vi "HPCNC CONTROL.vi"() -> ()   [LabVIEW 2014]
uses:
  SubVIs/HPCNC.lvlib
  <vilib>/Native 3D Graph/xcontrol/3DPC_SurfacePlot.xctl
  <vilib>/Instr/_visa.llb/VISA Configure Serial Port (Instr).vi
panel:
  out "New package":string
  in  "Enable":bool=TRUE
  in  "Stop":bool
  in  "Auto/Manual":bool=TRUE
  in  "Serial COM port":refnum<visa-resource-name>="COM4"
  in  "Pause":bool caption="Blank Button"
  in  "Start":bool caption="Blank Button"
  in  "RESET":bool caption="Blank Button"
  in  "HOME":bool caption="Blank Button"
  out "Check sum":bool=TRUE
  out "STATUS":string="Idle"
  out "Zm":string="0.000"
  out "Ym":string="-21.164"
  out "Xm":string="148.408"
  in  "Ys0":bool
  in  "Zs0":bool
  in  "Xs0":bool
  out "Za":string="0.000"
  out "Ya":string="0.000"
  out "Xa":string="0.000"
  in  "Enable Graph":bool
  in  "Clear Button":bool
  out "3D Graph":refnum<class "Base Datatype.lvclass">[](xcontrol)
  in  "JOG FR":i8(slide)=50 scale=0.0..100.0
  in  "Z-":bool caption="Blank Button"
  in  "Z+":bool caption="Blank Button"
  in  "Y-":bool caption="Blank Button"
  in  "Y+":bool caption="Blank Button"
  in  "X-":bool caption="Blank Button"
  in  "X+":bool caption="Blank Button"
  out "MANUAL":bool
  out "Current feed rate":string="0"
  in  "AUTO FR":i8(slide)=50 scale=0.0..100.0
  in  "G Code":string="G01X0Y0Z0F1000"
  in  "Send G code":bool caption="Blank Button"
  out "AUTOMATIC":bool=TRUE
  out "Receive data":string="\u001a0164<Id,MPos:148.408,-21.164,0.000,0.000,WPos:0.000,0.000,0.000,-3.500,Ln:0,F:0.,Fp:100,S:0.,Sp:100,SP:0,CL:0,MI:0,AS:1,JT:0,JM:0,Hi:0,AL:0,BC:458,CS:07\r\n"
  # "STATUS"
  # "MACHINE POSITION"
  # "X:"
  # "Y:"
  # "Z:"
  # "ABSOLUTE POSITION"
  # "X:"
  # "Y:"
  # "Z:"
  # "SIMULATION 3D"
  # "JOG"
  # "JOG FEED(%)"
  # "CMD:"
  # "CURRENT FEED RATE:"
  # "FEED RATE(%)"
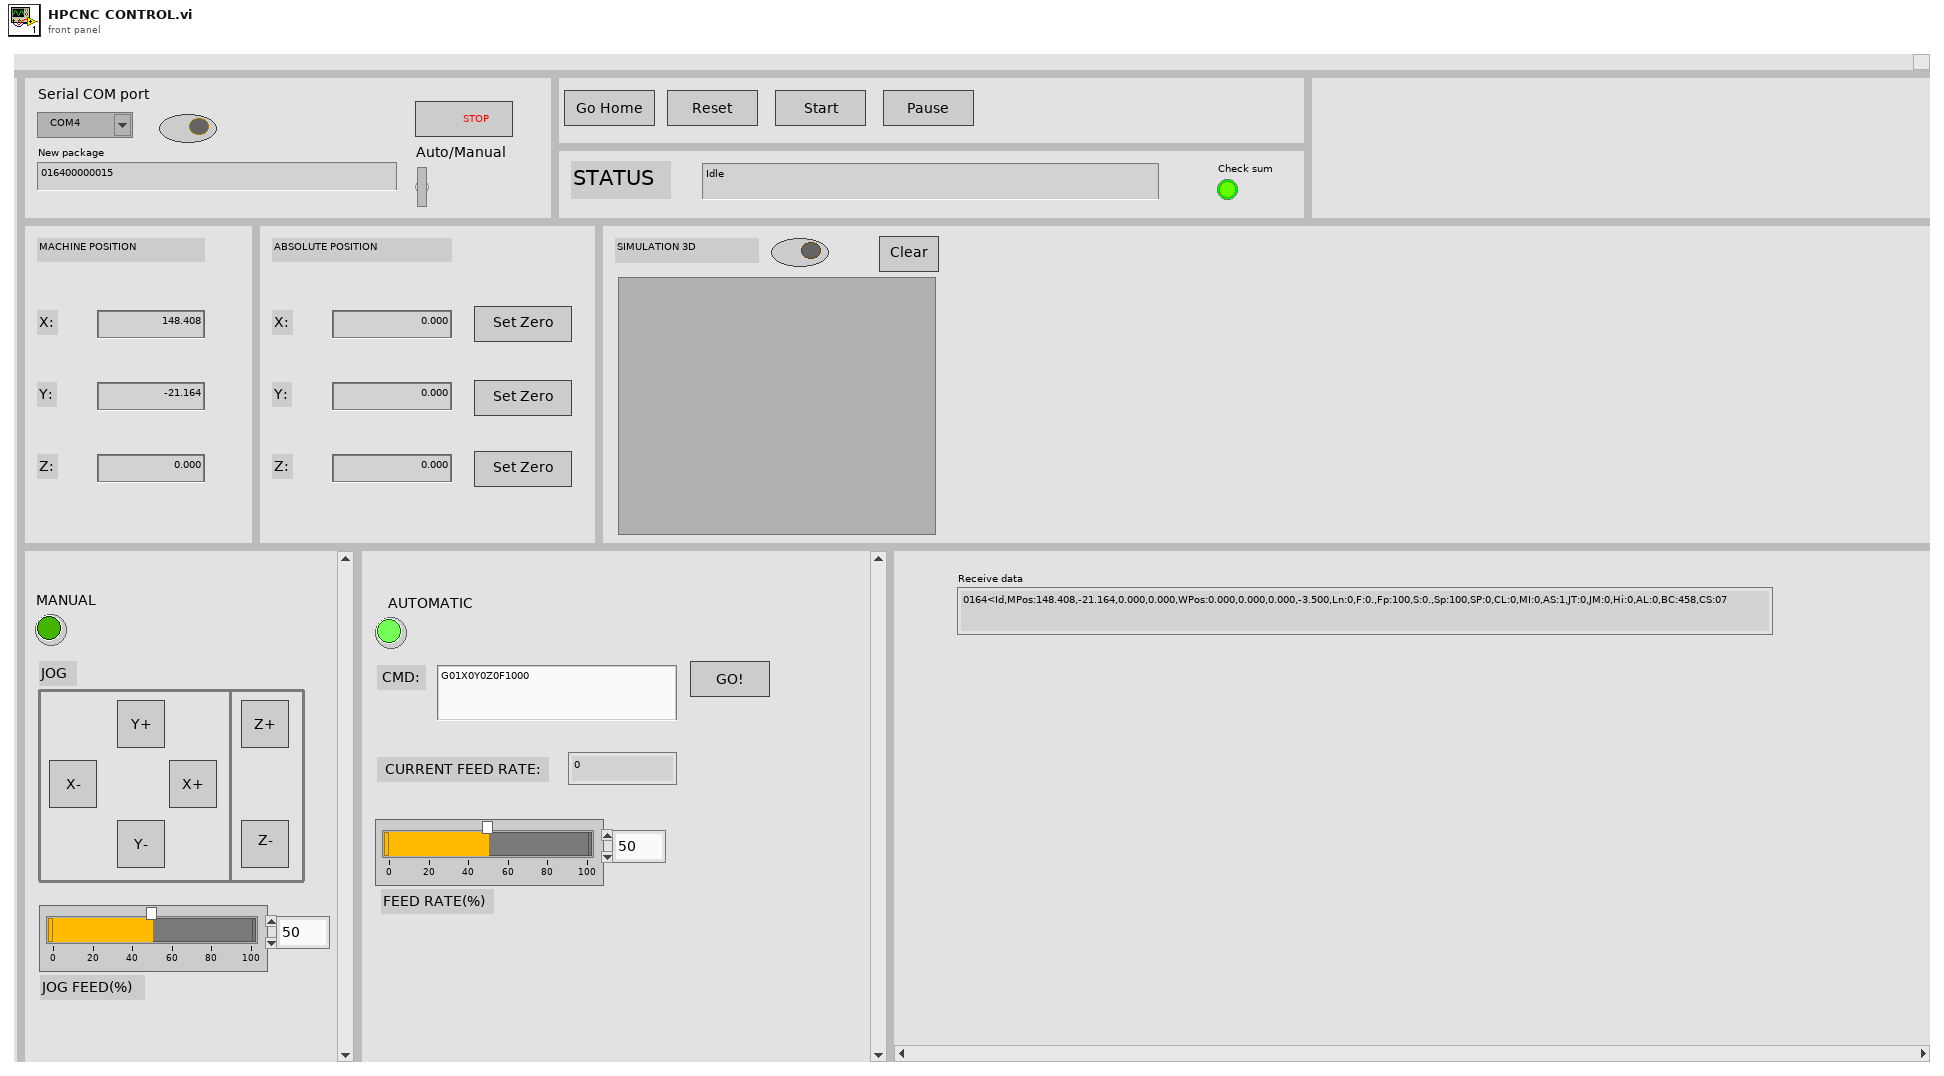
[diagram p1: front panel]
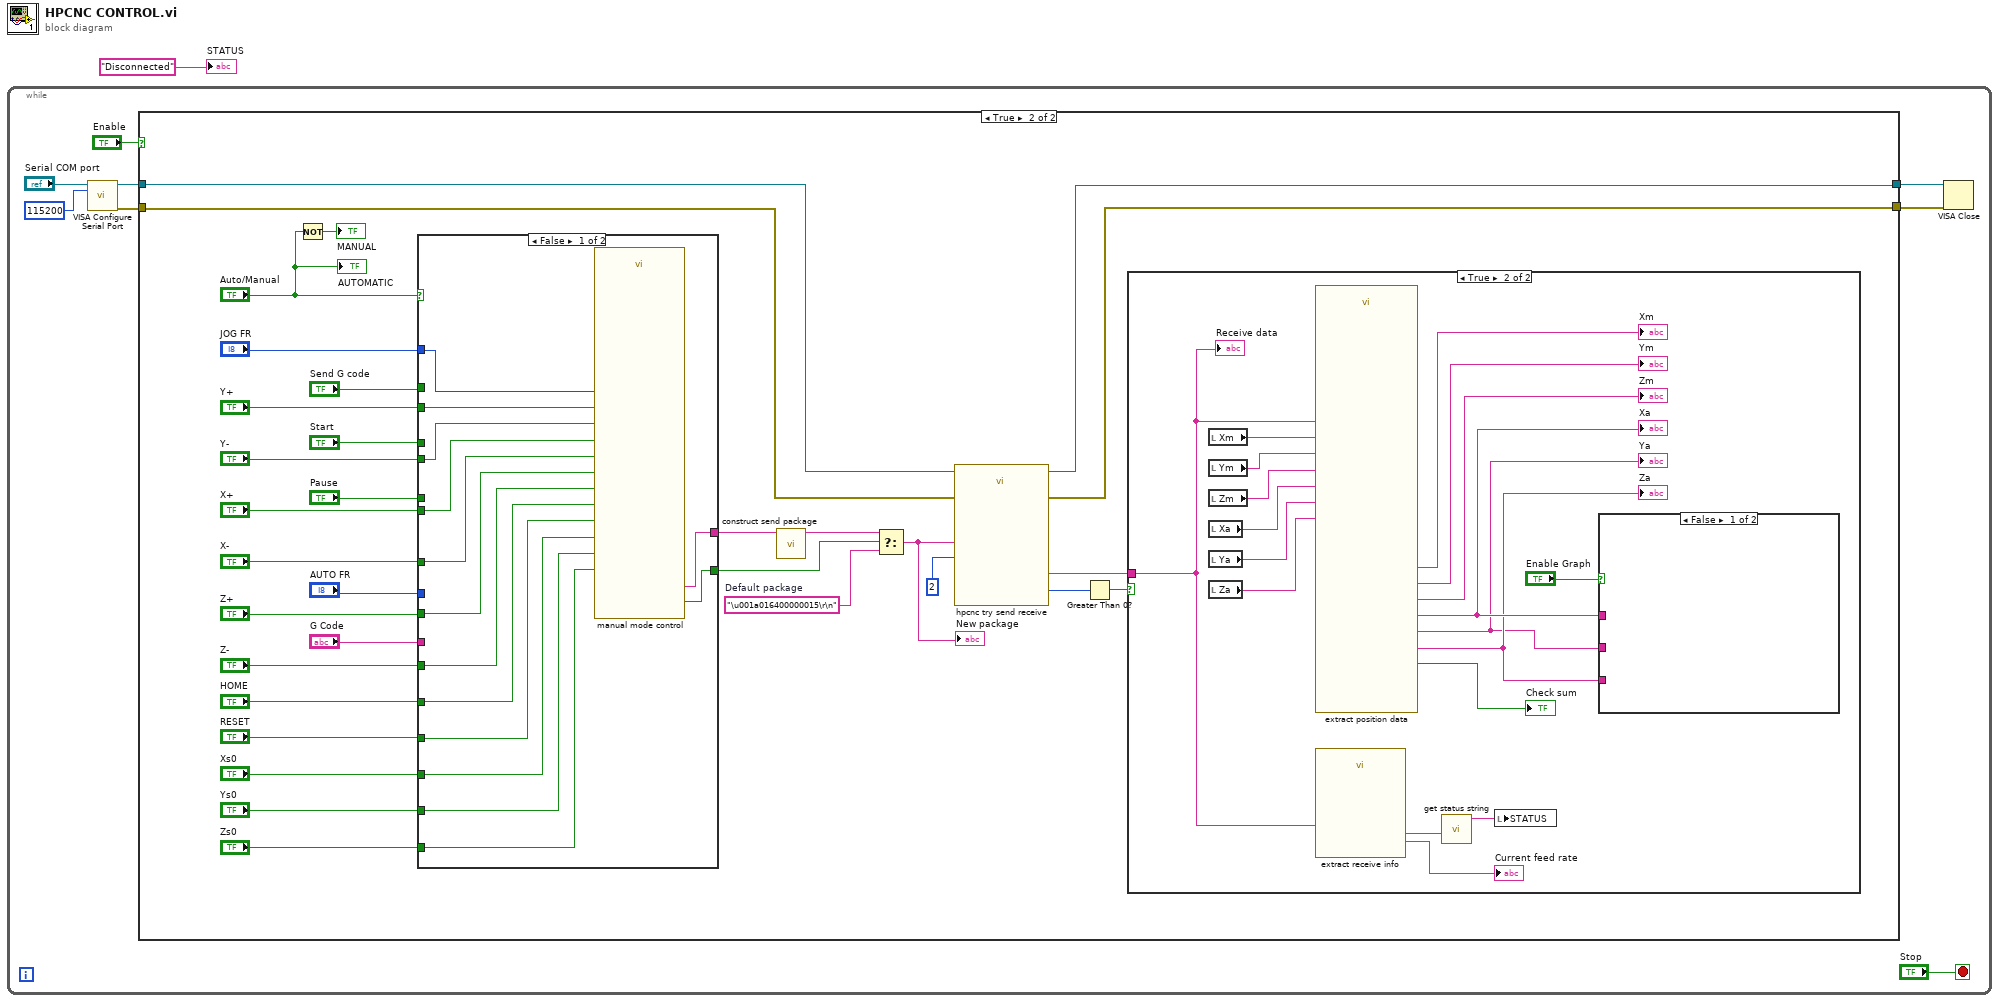
[diagram p0: block diagram]
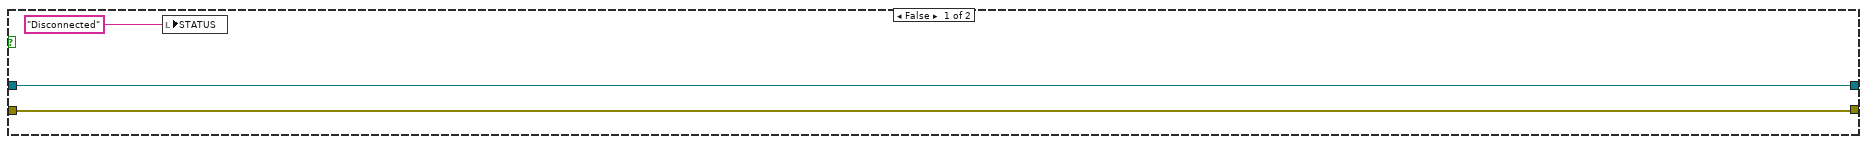
[diagram p2: hidden frame]
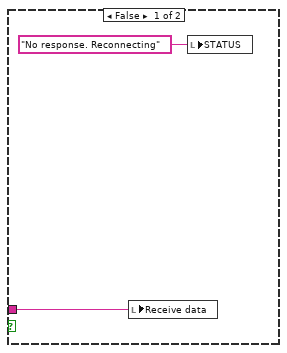
[diagram p3: hidden frame]
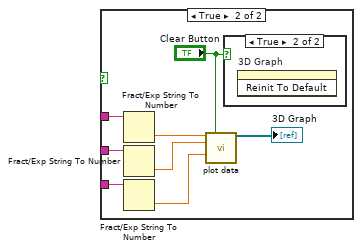
[diagram p4: hidden frame]
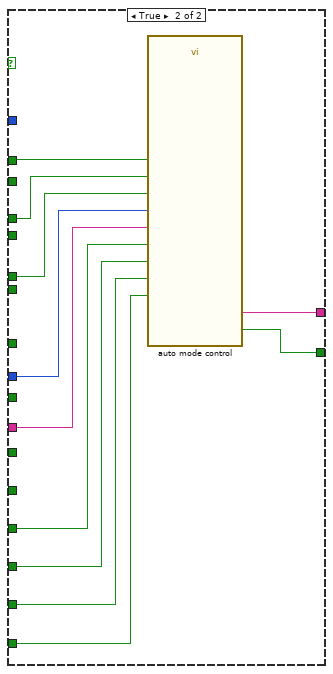
[diagram p6: hidden frame]
diagram:
  n1 = while {
    stop <- "Stop" stop-if-true
    n2 = call-poly "VISA Configure Serial Port"("VISA resource name"="Serial COM port", "baud rate (9600)"=u32 115200) -> ("VISA resource name out"=w5:refnum<visa-resource-name>, "error out"=w4:errorcluster)  [unwired: 12 in]
    n3 = case shown="True" "Enable" {
      tunnel: w5 -> [w12 w41]
      tunnel: w4 -> [w11 w44]
      tunnel: [w12 w43] -> w3
      tunnel: [w11 w42] -> w2
      frame False {
        n4 = local write "STATUS"("Disconnected" ("STATUS")) -> ()
      }
      frame True {
        w17 = "\u001a016400000015\r\n"  # Default package
        n5 = Not(x="Auto/Manual") -> (.not. x?=→"MANUAL":bool)
        n6 = case shown="False" "Auto/Manual" {
          tunnel: [w74 w97] -> w38
          tunnel: "Y+" -> [w80 _]
          tunnel: "Y-" -> [w79 _]
          tunnel: "X+" -> [w78 _]
          tunnel: "X-" -> [w86 _]
          tunnel: "Z+" -> [w85 _]
          tunnel: "Z-" -> [w77 _]
          tunnel: "HOME" -> [w76 _]
          tunnel: "JOG FR" -> [w84 _]
          tunnel: "Send G code" -> [_ w96]
          tunnel: "Start" -> [_ w90]
          tunnel: "Pause" -> [_ w89]
          tunnel: "AUTO FR" -> [_ w88]
          tunnel: "G Code" -> [_ w95]
          tunnel: "RESET" -> [w75 w94]
          tunnel: "Xs0" -> [w83 w93]
          tunnel: "Ys0" -> [w82 w92]
          tunnel: "Zs0" -> [w81 w91]
          tunnel: [w73 w87] -> w39
          frame False {
            n7 = call "manual mode control.vi"("X+"=w78, "Zs0"=w81, "X-"=w86, "Ys0"=w82, "Z+"=w85, "Y-"=w79, "Z-"=w77, "Y+"=w80, "HOME"=w76, "JOG FR"=w84, "RESET"=w75, "Xs0"=w83) -> ("Send command"=w74:string, "Valid command"=w73:bool)  [unwired: 6 in]
          }
          frame True {
            n8 = call "auto mode control.vi"("Pause"=w89, "Start"=w90, "Send GCode"=w96, "AUTO FR"=w88, "GCode"=w95, "RESET"=w94, "Xs0"=w93, "Ys0"=w92, "Zs0"=w91) -> ("Send command"=w97:string, "Valid command"=w87:bool)  [unwired: 5 in]
          }
        }
        n9 = call "construct send package.vi"("Send command"=w38) -> ("Send package"=w40:string)  [unwired: 8 in, 2 out]
        n10 = Select(t=w40, s=w39, f=w17) -> (s? t:f=w13:string)
        "New package" <- w13
        n11 = call "hpcnc try send receive.vi"("error in (no error)"=w44, "Max try number"=2, "Send package"=w13, "VISA Refnum in"=w41) -> ("error out"=w42:errorcluster, "Receive count"=w16:i32, "Receive package"=w15:string, "VISA Refnum out"=w43:refnum<visa-resource-name>)  [unwired: 4 in]
        n12 = Greater Than 0?(x=w16) -> (x > 0?=w14:bool)
        n13 = case shown="True" w14 {
          tunnel: w15 -> [w46 w49]
          frame False {
            n14 = local write "Receive data"(w46) -> ()
            n15 = local write "STATUS"("No response. Reconnecting" ("STATUS")) -> ()
          }
          frame True {
            n16 = local read "Xm"() -> (w57:string)
            n17 = local read "Ym"() -> (w56:string)
            n18 = local read "Zm"() -> (w55:string)
            n19 = local read "Xa"() -> (w54:string)
            n20 = local read "Ya"() -> (w53:string)
            n21 = local read "Za"() -> (w52:string)
            n22 = call "extract position data.vi"("Receive data"=w49, "Pre X_M"=w57, "Pre Y_M"=w56, "Pre Z_M"=w55, "Pre X_A"=w54, "Pre Y_A"=w53, "Pre Z_A"=w52) -> ("X_A"=w59:string, "Y_A"=w50:string, "Z_A"=w58:string, "X_M"=→"Xm":string, "Y_M"=→"Ym":string, "Z_M"=→"Zm":string, "CheckSumCorrect"=→"Check sum":bool)  [unwired: 10 in, 4 out]
            "Xa" <- w59
            "Ya" <- w50
            "Za" <- w58
            n23 = call "extract receive info.vi"("Receive data"=w49) -> ("STATUS"=w48:string, "Feed rate"=→"Current feed rate":string)  [unwired: 11 in, 2 out]
            n24 = call "get status string.vi"("Receive status"=w48) -> ("Status string"=w47:string)  [unwired: 10 in]
            n25 = local write "STATUS"(w47) -> ()
            n26 = case shown="False" "Enable Graph" {
              tunnel: w59 -> [_ w67]
              tunnel: w50 -> [_ w66]
              tunnel: w58 -> [_ w65]
              frame False {
              }
              frame True {
                n27 = Fract/Exp String To Number(string=w67) -> (number=w68:dbl)  [unwired: 3 in, 1 out]
                n28 = Fract/Exp String To Number(string=w66) -> (number=w69:dbl)  [unwired: 3 in, 1 out]
                n29 = Fract/Exp String To Number(string=w65) -> (number=w70:dbl)  [unwired: 3 in, 1 out]
                n30 = call "plot data.vi"("X"=w68, "Boolean"="Clear Button", "Y"=w69, "Z"=w70) -> ("plots out"=→"3D Graph":refnum<class "Base Datatype.lvclass">[])  [unwired: 8 in, 3 out]
                n31 = case shown="True" "Clear Button" {
                  frame False {
                  }
                  frame True {
                    n32 = invoke on="3D Graph" class="LabVIEW 3D Graph (strict)" method="Reinit To Default"() -> ()  [unwired: 3 in, 3 out]
                  }
                }
              }
            }
            "Receive data" <- w49
          }
        }
        "AUTOMATIC" <- "Auto/Manual"
      }
    }
    n33 = VISA Close(VISA resource name=w3, error in (no error)=w2) -> ()  [unwired: 1 out]
  }
  "STATUS" <- "Disconnected" ("STATUS")
